vi "InsertSelectRowTable.vi"(8 "エラー入力":errorcluster, 10 "挿入する指定行":i32, 11 "Tbl refnum":refnum<vi>) -> (0 "エラー出力":errorcluster, 3 "リファレンス出力":refnum<vi>)   [LabVIEW 2014]
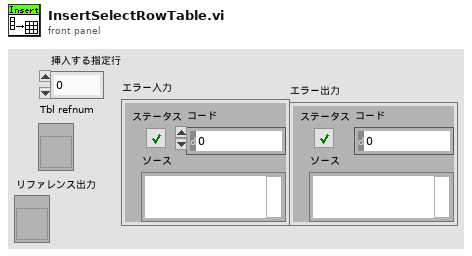
[diagram p1: front panel]
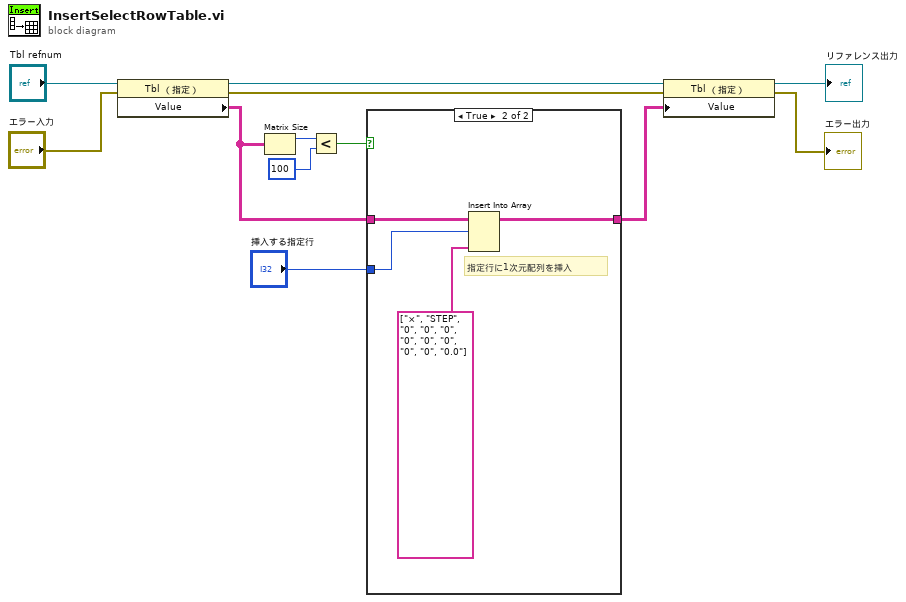
[diagram p0: block diagram]
diagram:
  n1 = property class="Tbl （指定）"(reference="Tbl refnum", error in="エラー入力") -> (reference out=w8:refnum<vi>, error out=w7:errorcluster, "Value"=w4:string[][])
  n2 = Matrix Size(0:w4) -> (1:w3:i32)  [unwired: 1 out]
  n3 = Less?(x=w3, y=100) -> (x < y?=w1:bool)
  n4 = case shown="TRUE" w1 {
    tunnel: "挿入する指定行" -> [_ w17]
    tunnel: [w13 w16] -> w5
    tunnel: w4 -> [w13 w14]
    frame False {
    }
    frame True {
      # "指定行に1次元配列を挿入"
      n5 = Insert Into Array(array=w14, index (row)=w17, new element=string[] ["×", "STEP", "0", "0", "0", "0", "0", "0", "0", "0", "0.0"] ("初期化配列")) -> (w16:string[][])  [unwired: 1 in]
    }
  }
  n6 = property class="Tbl （指定）"(reference=w8, error in=w7, "Value"=w5) -> (reference out=→"リファレンス出力":refnum<vi>, error out=→"エラー出力":errorcluster)
